vi "CS POLARIS BME DG.contents.vi"   [LabVIEW 2009, in "CS POLARIS BME DG.lvlib"]
uses:
  CS POLARIS BME DG.lvlib
types:
  T1 = typedef "CS POLARIS BME DG.lvlib/CS POLARIS BME DG.i attribute.ctl" = cluster{"Numeric":dbl, "DG_System":refnum<queue>, "UpdateTasks":refnum<queue>}
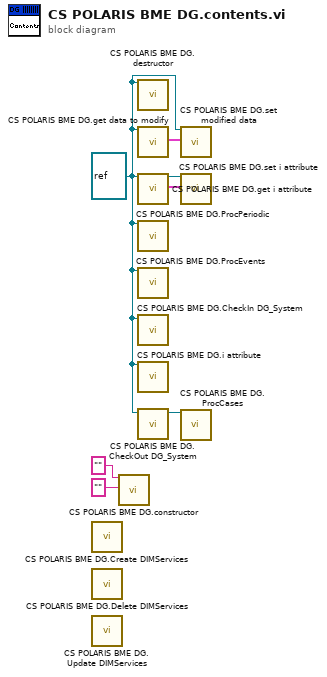
[diagram p0: block diagram]
diagram:
  w3 = refnum<vi> refnum ("i ref in")
  n1 = call "CS POLARIS BME DG.Create DIMServices.vi"() -> ()  [unwired: 10 in, 2 out]
  n2 = call "CS POLARIS BME DG.Delete DIMServices.vi"() -> ()  [unwired: 10 in, 2 out]
  n3 = call "CS POLARIS BME DG.Update DIMServices.vi"() -> ()  [unwired: 10 in, 2 out]
  n4 = call "CS POLARIS BME DG.constructor.vi"("name"="", "data in"="") -> ()  [unwired: 15 in, 3 out]
  n5 = call "CS POLARIS BME DG.destructor.vi"("i ref in"=w3) -> ()  [unwired: 18 in, 1 out]
  n6 = call "CS POLARIS BME DG.get data to modify.vi"("i ref in"=w3) -> ("i attribute"=w4:T1)  [unwired: 15 in, 3 out]
  n7 = call "CS POLARIS BME DG.get i attribute.vi"("i ref in"=w3) -> ("i ref out"=w1:refnum<vi>, "i attribute"=w5:T1)  [unwired: 16 in, 1 out]
  n8 = call "CS POLARIS BME DG.ProcPeriodic.vi"("i ref in"=w3) -> ()  [unwired: 16 in, 3 out]
  n9 = call "CS POLARIS BME DG.ProcEvents.vi"("i ref in"=w3) -> ()  [unwired: 17 in, 2 out]
  n10 = call "CS POLARIS BME DG.CheckIn DG_System.vi"("i ref in"=w3) -> ()  [unwired: 8 in, 2 out]
  n11 = call "CS POLARIS BME DG.i attribute.vi"("VI Refnum"=w3) -> ()  [unwired: 16 in, 3 out]
  n12 = call "CS POLARIS BME DG.CheckOut DG_System.vi"("i ref in"=w3) -> ("i ref out"=w2:refnum<vi>)  [unwired: 7 in, 3 out]
  n13 = call "CS POLARIS BME DG.set modified data.vi"("i ref in"=w3, "i attribute"=w4) -> ()  [unwired: 16 in, 2 out]
  n14 = call "CS POLARIS BME DG.set i attribute.vi"("i ref in"=w1, "i attribute"=w5) -> ()  [unwired: 16 in, 2 out]
  n15 = call "CS POLARIS BME DG.ProcCases.vi"("i ref in"=w2) -> ()  [unwired: 16 in, 3 out]
